vi "UPMAT.vi"(0 "功能":enum16{"物料上传", "绑定箱体"}(ring), 1 "物料名称":string, 2 "物料追溯码":string, 3 "工位追溯码":string, 4 "总成追溯码":string, 5 "错误输入":errorcluster, 6 "产品型号":string, 8 "设备型号":string) -> (14 "OK":bool, 19 "错误输出":errorcluster)   [LabVIEW 2019]
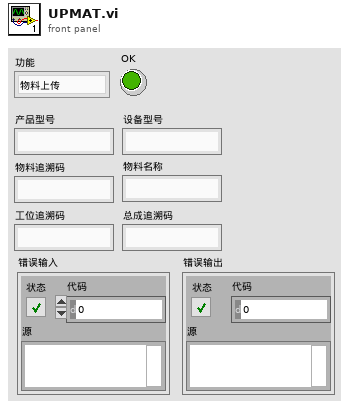
[diagram p1: front panel]
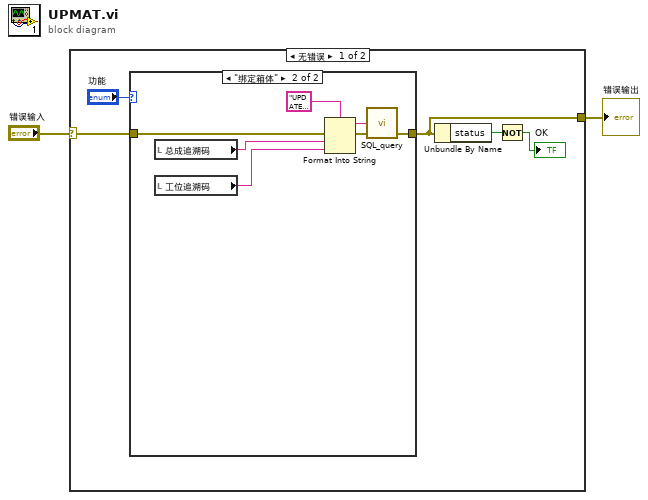
[diagram p0: block diagram]
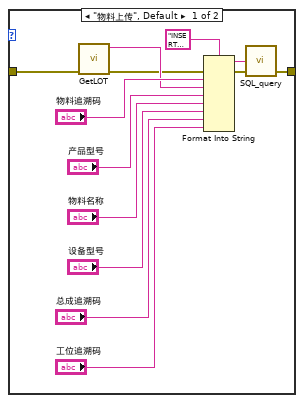
[diagram p2: hidden frame]
diagram:
  n1 = case shown="无错误" "错误输入" {
    selector: "错误输入" -> [w4 w28]
    tunnel: [w3 w28] -> w1
    frame No Error {
      n2 = case shown="\"绑定箱体\"" "功能" {
        tunnel: [w12 w27] -> w3
        tunnel: w4 -> [w10 w23]
        frame "物料上传", Default {
          n3 = call "GetLOT.vi"("错误输入"=w10) -> ("错误输出"=w9:errorcluster, "LOT"=w11:string)  [unwired: 8 in, 1 out]
          n4 = Format Into String(format string="INSERT INTO [SANLIserver].[dbo].[物料] (\n\t[物料追溯码],\n\t[生产编号],\n\t[产品型号],\n\t[物料名称],\n\t[设备型号],\n\t[总成追溯码],\n\t[工位追溯码]\n)VALUES\n\t(\n\t\tN'%s',\n\t\tN'%s',\n\t\tN'%s',\n\t\tN'%s',\n\t\tN'%s',\n\t\tN'%s',\n\t\tN'%s'\n\t)", error in=w9, "物料追溯码", w11, "产品型号", "物料名称", "设备型号", "总成追溯码", "工位追溯码") -> (resulting string=w13:string, error out=w8:errorcluster)  [unwired: 1 in]
          n5 = call "SQL_query.vi"("error in (no error)"=w8, "SQL query"=w13) -> ("error out"=w12:errorcluster)  [unwired: 1 in, 2 out]
        }
        frame "绑定箱体" {
          n6 = local read "总成追溯码"() -> (w25:string)
          n7 = local read "工位追溯码"() -> (w26:string)
          n8 = Format Into String(format string="UPDATE [SANLIserver].[dbo].[物料]\nSET [总成追溯码] = N'%s'\nWHERE\n\tdbo.[物料].[工位追溯码] = '%s'", error in=w23, w25, w26) -> (resulting string=w21:string, error out=w22:errorcluster)  [unwired: 1 in]
          n9 = call "SQL_query.vi"("error in (no error)"=w22, "SQL query"=w21) -> ("error out"=w27:errorcluster)  [unwired: 1 in, 2 out]
        }
      }
      n10 = Unbundle By Name(w3) -> ("status"=w6:bool)
      n11 = Not(x=w6) -> (.not. x?=→"OK":bool)
    }
    frame Error {
    }
  }
  "错误输出" <- w1
